vi "Write_Class_Relay_Board.vi"(8 "error in (no error)":errorcluster caption="entrée d'erreur (pas d'erreur)", 10 "Relay_Board (Default)":refnum<class "Class Relay_Board (Default).lvclass">, 11 "Class Relay_Board en entrée":refnum<class "Class Instrument Relay_Board.lvclass">) -> (0 "error out":errorcluster caption="sortie d'erreur", 3 "Class Relay_Board en Sortie":refnum<class "Class Instrument Relay_Board.lvclass">)   [LabVIEW 2020, in "Library Instrument & Equipement.lvlib" / "Library Instruments.lvlib" / "Class Instrument Relay_Board.lvclass"]
uses:
  Class Instrument Relay_Board.lvclass
  Relay_Board/Relay_Board (Default)/Class Relay_Board (Default).lvclass
  Class Instrument Relay_Board.lvclass/Class Instrument Relay_Board.ctl
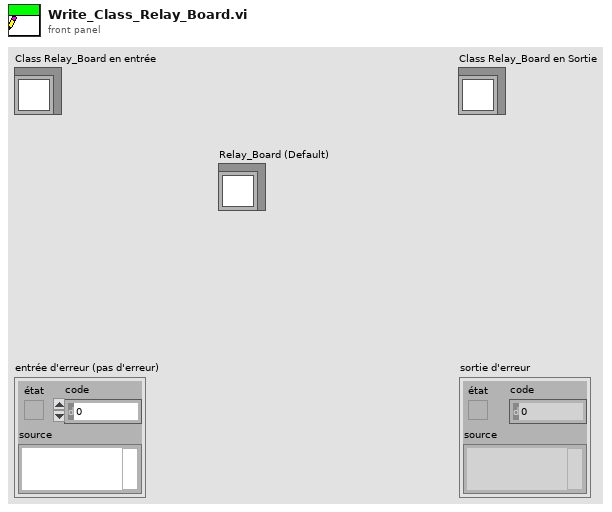
[diagram p1: front panel]
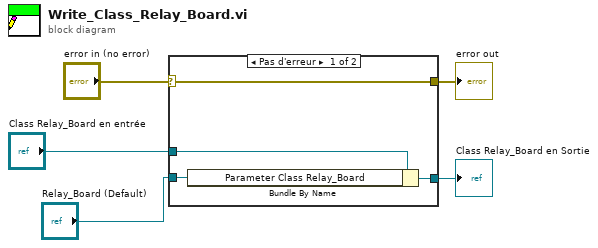
[diagram p0: block diagram]
diagram:
  n1 = case shown="Pas d'erreur" "error in (no error)" {
    selector: "error in (no error)" -> [w9 w10]
    tunnel: [w9 w10] -> w4
    tunnel: [w7 w11] -> w2
    tunnel: "Class Relay_Board en entrée" -> [w8 w11]
    tunnel: "Relay_Board (Default)" -> [w6 _]
    frame No Error {
      n2 = Bundle By Name(cluster=w8, "Parameter Class Relay_Board"=w6) -> (w7:refnum<class "Class Instrument Relay_Board.lvclass">)
    }
    frame Error {
    }
  }
  "error out" <- w4
  "Class Relay_Board en Sortie" <- w2
